vi "Analog_Ref_Num.vi"() -> (3 "Analog":T4)   [LabVIEW 2014]
uses:
  <vilib>/Rock Robotics/WPI/AnalogChannel/WPI_AnalogChannelDevRef.ctl
  <vilib>/Rock Robotics/SystemInterfaces/Typedef/FPGA_TypedefAnalogModule.ctl
  <vilib>/Rock Robotics/SystemInterfaces/AI/FPGA_AIChannel.ctl
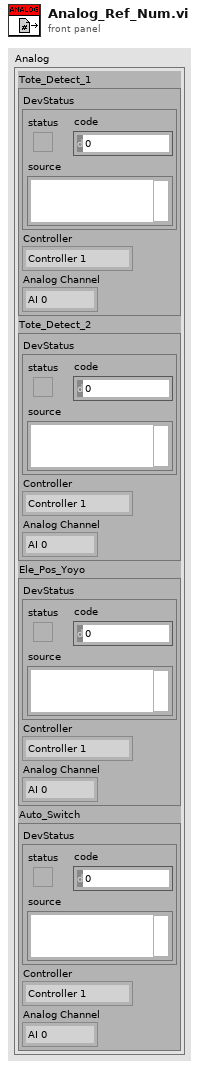
[diagram p1: front panel]
types:
  T1 = typedef "WPI_AnalogChannelDevRef.ctl" = cluster{"DevStatus":errorcluster, "Controller":T2, "Analog Channel":T3}
  T2 = typedef "FPGA_TypedefAnalogModule.ctl" = enum16{"Controller 1"}
  T3 = typedef "FPGA_AIChannel.ctl" = enum8{"AI 0", "AI 1", "AI 2", "AI 3", "AI MXP 0", "AI MXP 1", "AI MXP 2", "AI MXP 3", "Invalid"}
  T4 = cluster{"Tote_Detect_1":T1, "Tote_Detect_2":T1, "Ele_Pos_Yoyo":T1, "Auto_Switch":T1}
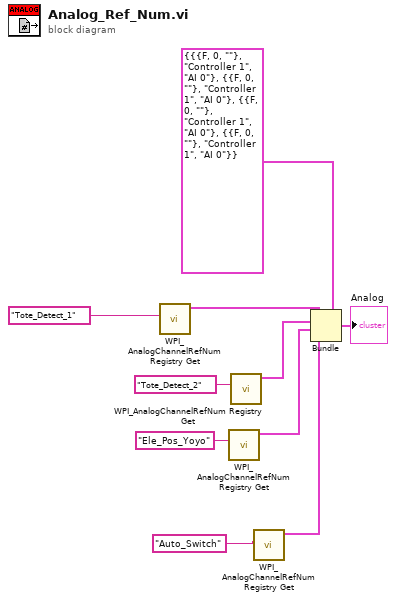
[diagram p0: block diagram]
diagram:
  n1 = call <vilib>:"WPI_AnalogChannelRefNum Registry Get.vi"("refnum name"="Tote_Detect_1") -> ("AIDeviceRef"=w4:T1)  [unwired: 9 in, 1 out]
  n2 = call <vilib>:"WPI_AnalogChannelRefNum Registry Get.vi"("refnum name"="Ele_Pos_Yoyo") -> ("AIDeviceRef"=w7:T1)  [unwired: 9 in, 1 out]
  n3 = call <vilib>:"WPI_AnalogChannelRefNum Registry Get.vi"("refnum name"="Tote_Detect_2") -> ("AIDeviceRef"=w8:T1)  [unwired: 9 in, 1 out]
  n4 = call <vilib>:"WPI_AnalogChannelRefNum Registry Get.vi"("refnum name"="Auto_Switch") -> ("AIDeviceRef"=w2:T1)  [unwired: 9 in, 1 out]
  n5 = Bundle(cluster=T4 {"Tote_Detect_1"={"DevStatus"={"status"=FALSE, "code"=0, "source"=""}, "Controller"=enum."Controller 1", "Analog Channel"=enum."AI 0"}, "Tote_Detect_2"={"DevStatus"={"status"=FALSE, "code"=0, "source"=""}, "Controller"=enum."Controller 1", "Analog Channel"=enum."AI 0"}, "Ele_Pos_Yoyo"={"DevStatus"={"status"=FALSE, "code"=0, "source"=""}, "Controller"=enum."Controller 1", "Analog Channel"=enum."AI 0"}, "Auto_Switch"={"DevStatus"={"status"=FALSE, "code"=0, "source"=""}, "Controller"=enum."Controller 1", "Analog Channel"=enum."AI 0"}}, "Tote_Detect_1"=w4, "Tote_Detect_2"=w8, "Ele_Pos_Yoyo"=w7, "Auto_Switch"=w2) -> (→"Analog":T4)
